vi "mxwScript_Cmnd2Str_createGrowableNode.vi"(8 "error in (no error)":errorcluster, 11 "data":variant) -> (0 "error out":errorcluster, 3 "outputString":string)   [LabVIEW 2020]
uses:
  codeGenAPISupport.llb/cgAPI_mxwScript_Wire_CreateGrowableNodeData.ctl
  codeGenAPISupport.llb/cgAPI_mxwScript_Wire_SupportedGrowableNodes.ctl
  codeGenAPISupport.llb/cgAPI_mxwScript_Wire_ArrayObjectPositionOptions.ctl
  codeGenAPISupport.llb/cgAPI_mxwScript_Wire_WireCreateSpaceData.ctl
  codeGenAPISupport.llb/cgAPI_mxwScript_Wire_GrowableNodeConnectToLocation.ctl
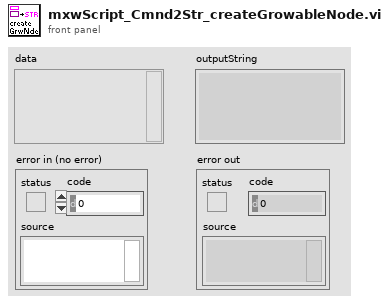
[diagram p1: front panel]
types:
  T1 = typedef "cgAPI_mxwScript_Wire_CreateGrowableNodeData.ctl" = cluster{"connectTo":string, "templateIndex":i32, "nodeName":string, "nodeType":T2, "nElements":i32, "positionOptions":T3, "wireSpace":T4, "connectToLocation":T5}
  T2 = typedef "cgAPI_mxwScript_Wire_SupportedGrowableNodes.ctl" = enum16{"IndexArray", "BuildArray", "DecimateArray", "InterleaveArray"}
  T3 = typedef "cgAPI_mxwScript_Wire_ArrayObjectPositionOptions.ctl" = enum16{"DoNotMove", "MoveTerminal", "MoveObject"}
  T4 = typedef "cgAPI_mxwScript_Wire_WireCreateSpaceData.ctl" = cluster{"nXPixelsPerWire":i32}
  T5 = typedef "cgAPI_mxwScript_Wire_GrowableNodeConnectToLocation.ctl" = enum16{"Top", "Terminal0"}
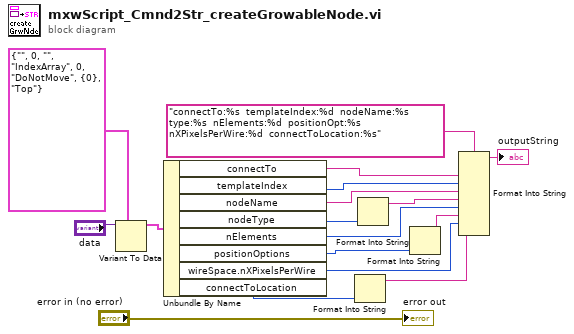
[diagram p0: block diagram]
diagram:
  n1 = Variant To Data(type=T1 {"connectTo"="", "templateIndex"=0, "nodeName"="", "nodeType"=enum."IndexArray", "nElements"=0, "positionOptions"=enum."DoNotMove", "wireSpace"={"nXPixelsPerWire"=0}, "connectToLocation"=enum."Top"} ("createGrowableNodeData"), Variant="data") -> (data=w16:T1)  [unwired: 1 in, 1 out]
  n2 = Unbundle By Name(w16) -> ("connectTo"=w8:string, "templateIndex"=w7:i32, "nodeName"=w6:string, "nodeType"=w9:T2, "nElements"=w4:i32, "positionOptions"=w10:T3, "wireSpace.nXPixelsPerWire"=w1:i32, "connectToLocation"=w11:T5)
  n3 = Format Into String(w11) -> (resulting string=w2:string)  [unwired: 3 in, 1 out]
  n4 = Format Into String(w9) -> (resulting string=w5:string)  [unwired: 3 in, 1 out]
  n5 = Format Into String(w10) -> (resulting string=w3:string)  [unwired: 3 in, 1 out]
  n6 = Format Into String(format string="connectTo:%s  templateIndex:%d  nodeName:%s  type:%s  nElements:%d  positionOpt:%s  nXPixelsPerWire:%d  connectToLocation:%s", w8, w7, w6, w5, w4, w3, w1, w2) -> (resulting string=→"outputString":string)  [unwired: 2 in, 1 out]
  "error out" <- "error in (no error)"
